vi "ParseArguments.vi"(8 "error in (no error)":errorcluster, 10 "CliArguments":string[](array[string]), 11 "ArgumentParser in":refnum<class "ArgumentParser.lvclass">) -> (0 "error out":errorcluster, 2 "ParsedData":T1, 3 "ArgumentParser out":refnum<class "ArgumentParser.lvclass">)   [LabVIEW 2022 SP3, in "ArgumentParser.lvlib" / "ArgumentParser.lvclass"]
uses:
  ArgumentParser.lvclass
  C:/Users/jakub/repos/gh/sw4sys/lv-argument-parser/PythonWrapper/Source/PythonWrapper/PythonWrapper.lvclass
  C:/Users/jakub/repos/gh/sw4sys/lv-argument-parser/ArgumentParser/Source/ArgparseWrapper/ArgparseWrapper.lvclass
  _ParsedData.ctl
  PythonWrapper/Source/PythonWrapper/PythonWrapper.lvclass/PythonWrapper.ctl
  ArgparseWrapper/ArgparseWrapper.lvclass/ArgparseWrapper.ctl
  ArgumentParser.lvclass/ArgumentParser.ctl
  PythonWrapper/Source/PythonWrapper/Read PythonSession.vi
  PythonWrapper/Source/PythonWrapper/Read ModulePath.vi
  ArgparseWrapper/Read FunctionParseArgs.vi
  Read Parser.vi
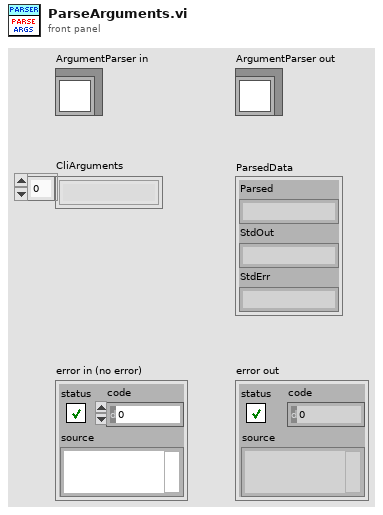
[diagram p1: front panel]
types:
  T1 = typedef "ArgumentParser.lvlib/ArgumentParser.lvclass/_ParsedData.ctl" = cluster{"Parsed":string, "StdOut":string, "StdErr":string}
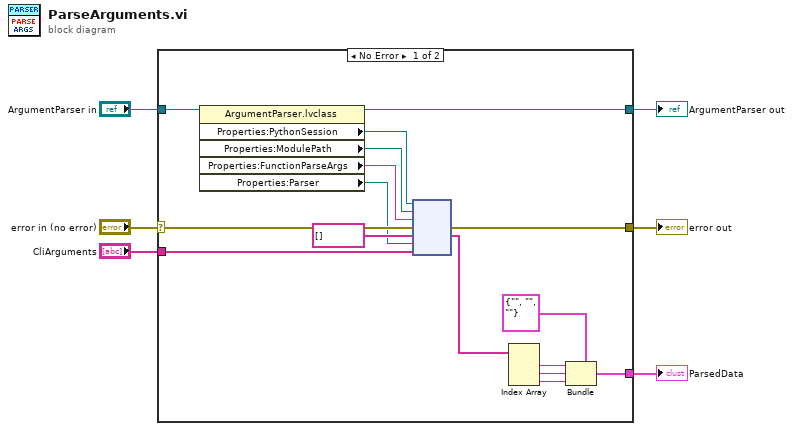
[diagram p0: block diagram]
diagram:
  n1 = case shown="No Error" "error in (no error)" {
    selector: "error in (no error)" -> [w22 w24]
    tunnel: [w21 w24] -> w5
    tunnel: [w11 w23] -> w3
    tunnel: "ArgumentParser in" -> [w20 w23]
    tunnel: "CliArguments" -> [w18 _]
    tunnel: [w13 _] -> w1
    frame No Error {
      n2 = property class="ArgumentParser.lvclass"(reference=w20) -> (reference out=w11:refnum<class "ArgumentParser.lvclass">, "Properties:PythonSession"=w9:refnum<k35>, "Properties:ModulePath"=w7:path, "Properties:FunctionParseArgs"=w8:string, "Properties:Parser"=w10:refnum<k38>)  [unwired: 1 in, 1 out]
      n3 = node(w9, w7, w8, w22, string[] [], w10, w18) -> (w21:errorcluster, w12:string[])  [unwired: 2 in, 3 out]
      n4 = Index Array(array=w12) -> (element #1=w16:string, element #2=w15:string, element #3=w14:string)  [unwired: 3 in]
      n5 = Bundle(cluster=T1 {"Parsed"="", "StdOut"="", "StdErr"=""} ("ParsedData"), "Parsed"=w16, "StdOut"=w15, "StdErr"=w14) -> (w13:T1)
    }
    frame Error {
    }
  }
  "error out" <- w5
  "ArgumentParser out" <- w3
  "ParsedData" <- w1
